vi "GetParam.vi"(8 "error in (no error)":errorcluster caption="entrée d'erreur (pas d'erreur)", 11 "maxabs_scale.lvclass":refnum<class "maxabs_scale.lvclass">) -> (0 "error out":errorcluster caption="sortie d'erreur", 2 "maxabs_scale":cluster{"axis":i32, "copy":bool}={"axis"=0, "copy"=TRUE}, 3 "maxabs_scale.lvclass":refnum<class "maxabs_scale.lvclass">)   [LabVIEW 2020, in "maxabs_scale.lvclass"]
doc: "Get Parameters"
uses:
  maxabs_scale.lvclass
  maxabs_scale.lvclass/maxabs_scale.ctl
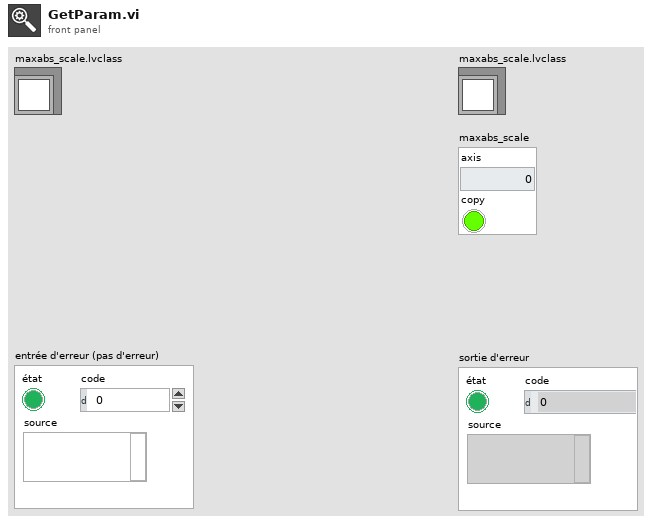
[diagram p1: front panel]
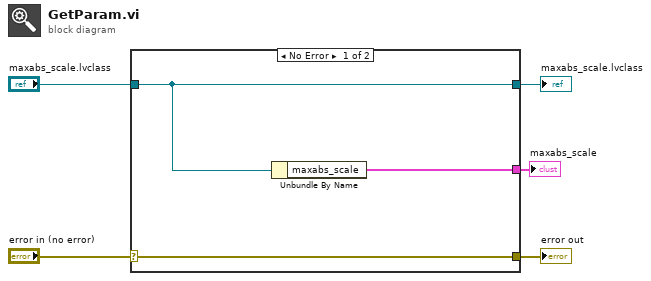
[diagram p0: block diagram]
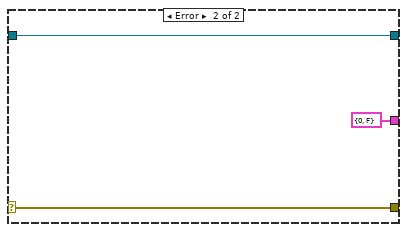
[diagram p2: hidden frame]
diagram:
  n1 = case shown="No Error" "error in (no error)" {
    selector: "error in (no error)" -> [w8 w10]
    tunnel: [w8 w10] -> w4
    tunnel: [w7 w11] -> w2
    tunnel: "maxabs_scale.lvclass" -> [w7 w11]
    tunnel: [w6 cluster{"axis":i32, "copy":bool} {"axis"=0, "copy"=FALSE} ("maxabs_scale")] -> w1
    frame No Error {
      n2 = Unbundle By Name(w7) -> ("maxabs_scale"=w6:cluster{"axis":i32, "copy":bool})
    }
    frame Error {
    }
  }
  "error out" <- w4
  "maxabs_scale.lvclass" <- w2
  "maxabs_scale" <- w1
